vi "Get Addresses.vi"() -> (2 "Addresses":string[](array[string]), 3 "IP Addresses":T1[](array[typedef]) {"MAC U64" format="%012x"; "Mask" format="%08x"; "Address" format="%08x"})   [LabVIEW 2021, in "Networking_CIF_U.lvlib"]
doc: "Get the IPV4 address and subnet mask, the MAC address, and the resource description for all adaptors on the system. \n\nThe address list is filtered to only include valid IPV4 addresses with a valid MAC address. \n\nThis uses standard Windows and Linux system calls and parses the response."
uses:
  Networking_CIF_U.lvlib
  Typedef/IPV4 Address.ctl
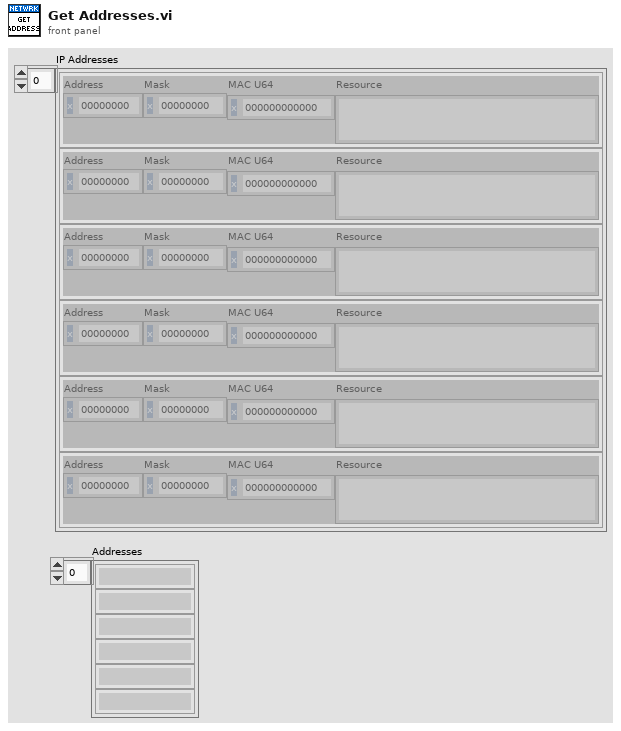
[diagram p1: front panel]
types:
  T1 = typedef "Networking_CIF_U.lvlib/IPV4 Address.ctl" = cluster{"Address":u32, "Mask":u32, "MAC U64":u64, "Resource":string}
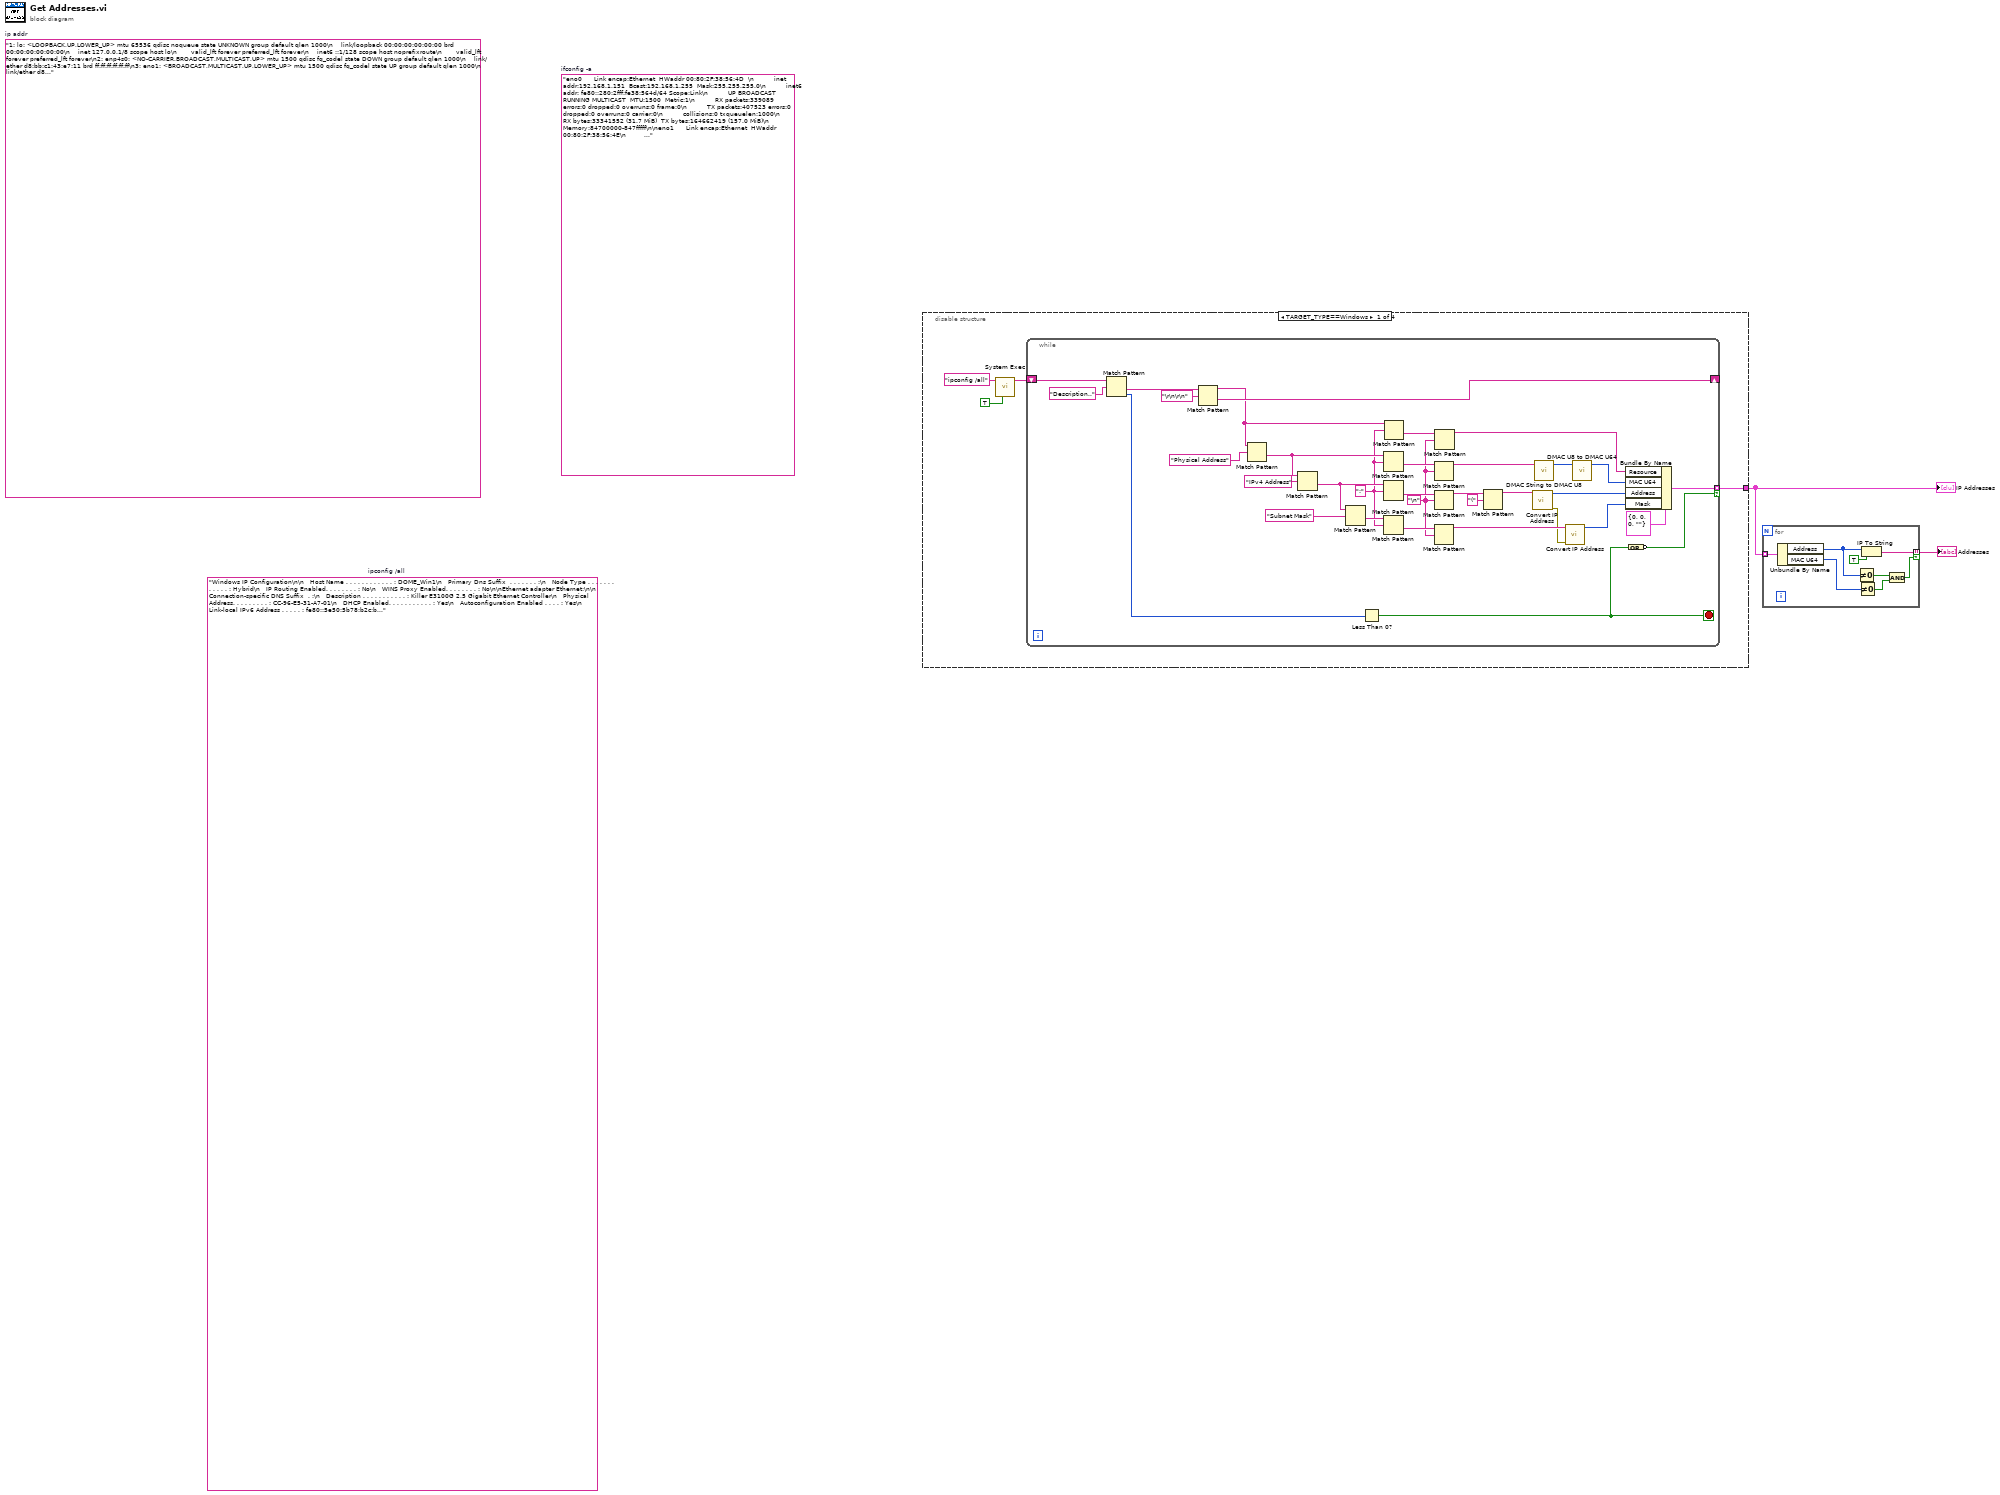
[diagram p0: block diagram]
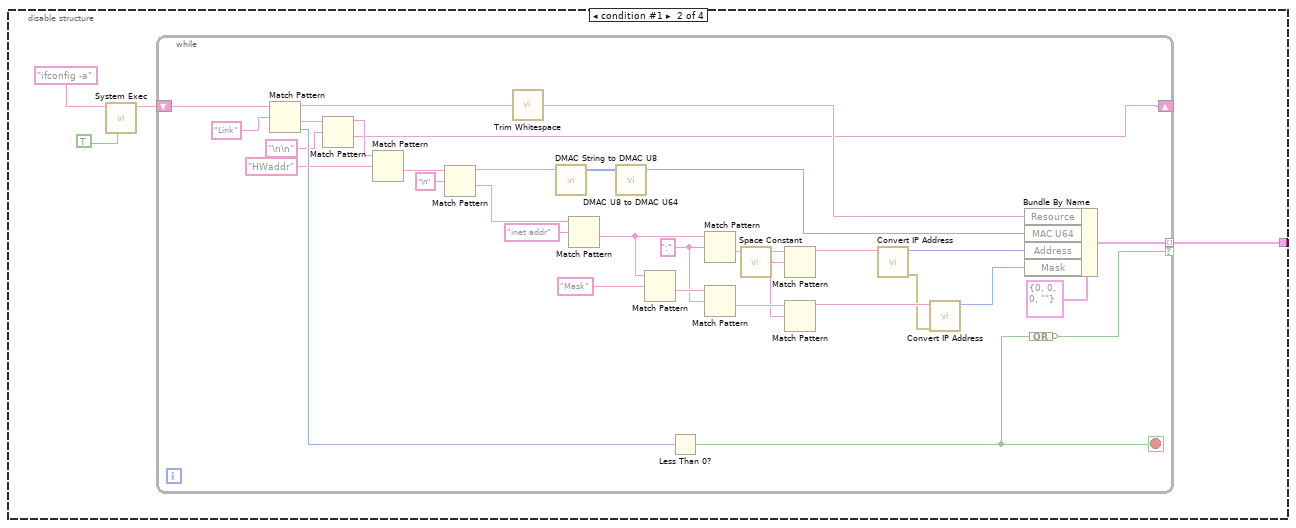
[diagram p2: hidden frame]
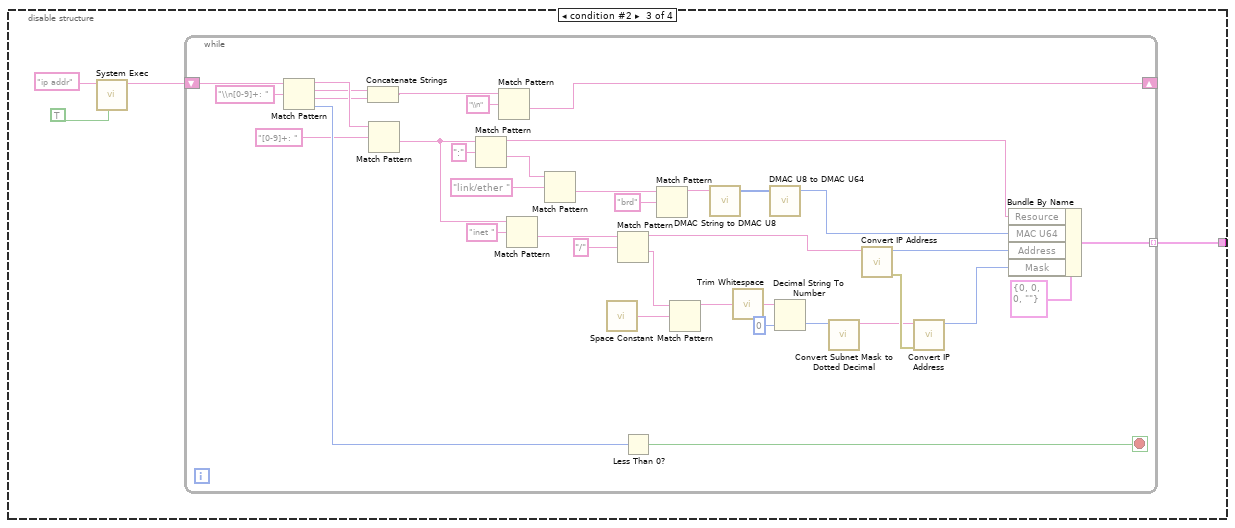
[diagram p3: hidden frame]
diagram:
  (unwired) "Windows IP Configuration\n\n   Host Name . . . . . . . . . . . . : DOME_Win1\n   Primary Dns Suffix  . . . . . . . :\n   Node Type . . . . . . . . . . . . : Hybrid\n   IP Routing Enabled. . . . . . . . : No\n   WINS Proxy Enabled. . . . . . . . : No\n\nEthernet adapter Ethernet:\n\n   Connection-specific DNS Suffix  . :\n   Description . . . . . . . . . . . : Killer E3100G 2.5 Gigabit Ethernet Controller\n   Physical Address. . . . . . . . . : CC-96-E5-31-A7-01\n   DHCP Enabled. . . . . . . . . . . : Yes\n   Autoconfiguration Enabled . . . . : Yes\n   Link-local IPv6 Address . . . . . : fe80::5e50:5b78:b2c:bb23%16(Preferred)\n   IPv4 Address. . . . . . . . . . . : 192.168.1.118(Preferred)\n   Subnet Mask . . . . . . . . . . . : 255.255.255.0\n   Lease Obtained. . . . . . . . . . : Monday, December 1, 2025 1:30:17 PM\n   Lease Expires . . . . . . . . . . : Sunday, January 10, 2162 1:38:58 AM\n   Default Gateway . . . . . . . . . : 192.168.1.1\n   DHCP Server . . . . . . . . . . . : 192.168.1.1\n   DHCPv6 IAID . . . . . . . . . . . : 114071269\n   DHCPv6 Client DUID. . . . . . . . : 00-01-00-01-2C-F9-5E-4C-CC-96-E5-31-A7-01\n   DNS Servers . . . . . . . . . . . : 208.67.222.123\n                                       208.67.220.123\n   NetBIOS over Tcpip. . . . . . . . : Enabled\n\nWireless LAN adapter Wi-Fi:\n\n   Media State . . . . . . . . . . . : Media disconnected\n   Connection-specific DNS Suffix  . :\n   Description . . . . . . . . . . . : Killer(R) Wi-Fi 6E AX1675i 160MHz Wireless Network Adapter (211NGW)\n   Physical Address. . . . . . . . . : 8C-17-59-A9-DC-15\n   DHCP Enabled. . . . . . . . . . . : Yes\n   Autoconfiguration Enabled . . . . : Yes\n\nWireless LAN adapter Local Area Connection* 1:\n\n   Media State . . . . . . . . . . . : Media disconnected\n   Connection-specific DNS Suffix  . :\n   Description . . . . . . . . . . . : Microsoft Wi-Fi Direct Virtual Adapter\n   Physical Address. . . . . . . . . : 8C-17-59-A9-DC-16\n   DHCP Enabled. . . . . . . . . . . : Yes\n   Autoconfiguration Enabled . . . . : Yes\n\nWireless LAN adapter Local Area Connection* 2:\n\n   Media State . . . . . . . . . . . : Media disconnected\n   Connection-specific DNS Suffix  . :\n   Description . . . . . . . . . . . : Microsoft Wi-Fi Direct Virtual Adapter #2\n   Physical Address. . . . . . . . . : 8E-17-59-A9-DC-15\n   DHCP Enabled. . . . . . . . . . . : Yes\n   Autoconfiguration Enabled . . . . : Yes\n\nEthernet adapter VMware Network Adapter VMnet1:\n\n   Connection-specific DNS Suffix  . :\n   Description . . . . . . . . . . . : VMware Virtual Ethernet Adapter for VMnet1\n   Physical Address. . . . . . . . . : 00-50-56-C0-00-01\n   DHCP Enabled. . . . . . . . . . . : Yes\n   Autoconfiguration Enabled . . . . : Yes\n   Link-local IPv6 Address . . . . . : fe80::dc23:c337:5224:768b%14(Preferred)\n   IPv4 Address. . . . . . . . . . . : 192.168.116.1(Preferred)\n   Subnet Mask . . . . . . . . . . . : 255.255.255.0\n   Lease Obtained. . . . . . . . . . : Monday, December 1, 2025 1:30:14 PM\n   Lease Expires . . . . . . . . . . : Wednesday, December 3, 2025 7:28:46 PM\n   Default Gateway . . . . . . . . . :\n   DHCP Server . . . . . . . . . . . : 192.168.116.254\n   DHCPv6 IAID . . . . . . . . . . . : 822104150\n   DHCPv6 Client DUID. . . . . . . . : 00-01-00-01-2C-F9-5E-4C-CC-96-E5-31-A7-01\n   NetBIOS over Tcpip. . . . . . . . : Enabled\n\nEthernet adapter VMware Network Adapter VMnet8:\n\n   Connection-specific DNS Suffix  . :\n   Description . . . . . . . . . . . : VMware Virtual Ethernet Adapter for VMnet8\n   Physical Address. . . . . . . . . : 00-50-56-C0-00-08\n   DHCP Enabled. . . . . . . . . . . : Yes\n   Autoconfiguration Enabled . . . . : Yes\n   Link-local IPv6 Address . . . . . : fe80::ac10:2aab:234a:a114%4(Preferred)\n   IPv4 Address. . . . . . . . . . . : 192.168.153.1(Preferred)\n   Subnet Mask . . . . . . . . . . . : 255.255.255.0\n   Lease Obtained. . . . . . . . . . : Monday, December 1, 2025 1:30:17 PM\n   Lease Expires . . . . . . . . . . : Wednesday, December 3, 2025 7:28:46 PM\n   Default Gateway . . . . . . . . . :\n   DHCP Server . . . . . . . . . . . : 192.168.153.254\n   DHCPv6 IAID . . . . . . . . . . . : 855658582\n   DHCPv6 Client DUID. . . . . . . . : 00-01-00-01-2C-F9-5E-4C-CC-96-E5-31-A7-01\n   Primary WINS Server . . . . . . . : 192.168.153.2\n   NetBIOS over Tcpip. . . . . . . . : Enabled\n\nEthernet adapter Bluetooth Network Connection:\n\n   Media State . . . . . . . . . . . : Media disconnected\n   Connection-specific DNS Suffix  . :\n   Description . . . . . . . . . . . : Bluetooth Device (Personal Area Network)\n   Physical Address. . . . . . . . . : 8C-17-59-A9-DC-19\n   DHCP Enabled. . . . . . . . . . . : Yes\n   Autoconfiguration Enabled . . . . : Yes"  # ipconfig /all
  (unwired) "eno0      Link encap:Ethernet  HWaddr 00:80:2F:38:56:4D  \n          inet addr:192.168.1.151  Bcast:192.168.1.255  Mask:255.255.255.0\n          inet6 addr: fe80::280:2fff:fe38:564d/64 Scope:Link\n          UP BROADCAST RUNNING MULTICAST  MTU:1500  Metric:1\n          RX packets:339089 errors:0 dropped:0 overruns:0 frame:0\n          TX packets:407523 errors:0 dropped:0 overruns:0 carrier:0\n          collisions:0 txqueuelen:1000\n          RX bytes:33341552 (31.7 MiB)  TX bytes:164662419 (157.0 MiB)\n          Memory:84700000-847fffff\n\neno1      Link encap:Ethernet  HWaddr 00:80:2F:38:56:4E\n          UP BROADCAST MULTICAST  MTU:1500  Metric:1\n          RX packets:0 errors:0 dropped:0 overruns:0 frame:0\n          TX packets:0 errors:0 dropped:0 overruns:0 carrier:0\n          collisions:0 txqueuelen:1000\n          RX bytes:0 (0.0 B)  TX bytes:0 (0.0 B)\n          Memory:84a00000-84afffff\n\nenp19s0f0 Link encap:Ethernet  HWaddr 08:C0:EB:46:0E:84\n          UP BROADCAST MULTICAST  MTU:1500  Metric:1\n          RX packets:0 errors:0 dropped:0 overruns:0 frame:0\n          TX packets:0 errors:0 dropped:0 overruns:0 carrier:0\n          collisions:0 txqueuelen:1000\n          RX bytes:0 (0.0 B)  TX bytes:0 (0.0 B)\n\nenp19s0f1 Link encap:Ethernet  HWaddr 08:C0:EB:46:0E:85\n          inet addr:192.168.12.2  Bcast:192.168.12.255  Mask:255.255.255.0\n          inet6 addr: fe80::ac0:ebff:fe46:e85/64 Scope:Link\n          UP BROADCAST RUNNING MULTICAST  MTU:1500  Metric:1\n          RX packets:283252 errors:0 dropped:0 overruns:0 frame:0\n          TX packets:61426 errors:0 dropped:0 overruns:0 carrier:0\n          collisions:0 txqueuelen:1000\n          RX bytes:355620193 (339.1 MiB)  TX bytes:16833550 (16.0 MiB)\n\nlo        Link encap:Local Loopback\n          inet addr:127.0.0.1  Mask:255.0.0.0\n          inet6 addr: ::1/128 Scope:Host\n          UP LOOPBACK RUNNING  MTU:65536  Metric:1\n          RX packets:134558 errors:0 dropped:0 overruns:0 frame:0\n          TX packets:134558 errors:0 dropped:0 overruns:0 carrier:0\n          collisions:0 txqueuelen:1000\n          RX bytes:11949346 (11.3 MiB)  TX bytes:11949346 (11.3 MiB)"  # ifconfig -a
  (unwired) "1: lo: <LOOPBACK,UP,LOWER_UP> mtu 65536 qdisc noqueue state UNKNOWN group default qlen 1000\n    link/loopback 00:00:00:00:00:00 brd 00:00:00:00:00:00\n    inet 127.0.0.1/8 scope host lo\n       valid_lft forever preferred_lft forever\n    inet6 ::1/128 scope host noprefixroute\n       valid_lft forever preferred_lft forever\n2: enp4s0: <NO-CARRIER,BROADCAST,MULTICAST,UP> mtu 1500 qdisc fq_codel state DOWN group default qlen 1000\n    link/ether d8:bb:c1:43:e7:11 brd ff:ff:ff:ff:ff:ff\n3: eno1: <BROADCAST,MULTICAST,UP,LOWER_UP> mtu 1500 qdisc fq_codel state UP group default qlen 1000\n    link/ether d8:bb:c1:43:e7:10 brd ff:ff:ff:ff:ff:ff\n    altname enp0s31f6\n    inet 192.168.1.242/24 brd 192.168.1.255 scope global noprefixroute eno1\n       valid_lft forever preferred_lft forever\n    inet6 fe80::dabb:c1ff:fe43:e710/64 scope link\n       valid_lft forever preferred_lft forever\n4: enp23s0f0np0: <NO-CARRIER,BROADCAST,MULTICAST,UP> mtu 1500 qdisc mq state DOWN group default qlen 1000\n    link/ether 04:3f:72:bd:14:a2 brd ff:ff:ff:ff:ff:ff\n5: enp23s0f1np1: <NO-CARRIER,BROADCAST,MULTICAST,UP> mtu 1500 qdisc mq state DOWN group default qlen 1000\n    link/ether 04:3f:72:bd:14:a3 brd ff:ff:ff:ff:ff:ff\n7: docker0: <NO-CARRIER,BROADCAST,MULTICAST,UP> mtu 1500 qdisc noqueue state DOWN group default\n    link/ether 8a:5f:4f:9d:9b:22 brd ff:ff:ff:ff:ff:ff\n    inet 172.17.0.1/16 brd 172.17.255.255 scope global docker0\n       valid_lft forever preferred_lft forever\n    inet6 fe80::885f:4fff:fe9d:9b22/64 scope link\n       valid_lft forever preferred_lft forever\n2022: br-b6147a662842: <BROADCAST,MULTICAST,UP,LOWER_UP> mtu 1500 qdisc noqueue state UP group default\n    link/ether e6:81:36:eb:4b:75 brd ff:ff:ff:ff:ff:ff\n    inet 172.18.0.1/16 brd 172.18.255.255 scope global br-b6147a662842\n       valid_lft forever preferred_lft forever\n    inet6 fe80::e481:36ff:feeb:4b75/64 scope link\n       valid_lft forever preferred_lft forever\n2025: veth8e9c1bb@if2: <BROADCAST,MULTICAST,UP,LOWER_UP> mtu 1500 qdisc noqueue master br-b6147a662842 state UP group default\n    link/ether 66:7b:84:4d:96:ba brd ff:ff:ff:ff:ff:ff link-netnsid 0\n    inet6 fe80::647b:84ff:fe4d:96ba/64 scope link\n       valid_lft forever preferred_lft forever\n2026: veth719d540@if2: <BROADCAST,MULTICAST,UP,LOWER_UP> mtu 1500 qdisc noqueue master br-b6147a662842 state UP group default\n    link/ether 4e:3e:af:11:6f:2c brd ff:ff:ff:ff:ff:ff link-netnsid 1\n    inet6 fe80::4c3e:afff:fe11:6f2c/64 scope link\n       valid_lft forever preferred_lft forever\n2034: br-e29f2d474aae: <NO-CARRIER,BROADCAST,MULTICAST,UP> mtu 1500 qdisc noqueue state DOWN group default\n    link/ether 76:6d:e5:b8:89:b4 brd ff:ff:ff:ff:ff:ff\n    inet 172.19.0.1/16 brd 172.19.255.255 scope global br-e29f2d474aae\n       valid_lft forever preferred_lft forever\n    inet6 fe80::746d:e5ff:feb8:89b4/64 scope link\n       valid_lft forever preferred_lft forever"  # ip addr
  n1 = disable-structure shown="TARGET_TYPE==Windows" {
    disable-tunnel: [w3 w41 w79 _] -> w2
    frame condition #0 (active) {
      n2 = call <vilib>:"System Exec.vi"("run minimized? (F)"=TRUE, "command line"="ipconfig /all") -> ("standard output"=w4:string)  [unwired: 6 in, 3 out]
      n3 = while {
        shift-right: [w12] -> _
        shift-left: w4 -> [w17]
        tunnel: [w28] -> w3 mode=indexing if=w27
        stop <- w29 stop-if-true
        w9 = "\n"
        w10 = ":" ("regular expression")
        n4 = Match Pattern(string=w17, regular expression="Description..") -> (after substring=w14:string, offset past match=w15:i32)  [unwired: 1 in, 2 out]
        n5 = Match Pattern(string=w14, regular expression="\r\n\r\n") -> (before substring=w8:string, after substring=w12:string)  [unwired: 1 in, 2 out]
        n6 = Match Pattern(string=w8, regular expression="Physical Address") -> (after substring=w24:string)  [unwired: 1 in, 3 out]
        n7 = Match Pattern(string=w24, regular expression="IPv4 Address") -> (after substring=w38:string)  [unwired: 1 in, 3 out]
        n8 = Match Pattern(string=w38, regular expression="Subnet Mask") -> (after substring=w37:string)  [unwired: 1 in, 3 out]
        n9 = Less Than 0?(x=w15) -> (x < 0?=w29:bool)
        n10 = Match Pattern(string=w24, regular expression=w10) -> (after substring=w25:string)  [unwired: 1 in, 3 out]
        n11 = Match Pattern(string=w38, regular expression=w10) -> (after substring=w36:string)  [unwired: 1 in, 3 out]
        n12 = Match Pattern(string=w37, regular expression=w10) -> (after substring=w35:string)  [unwired: 1 in, 3 out]
        n13 = Match Pattern(string=w8, regular expression=w10) -> (after substring=w11:string)  [unwired: 1 in, 3 out]
        n14 = Match Pattern(string=w25, regular expression=w9) -> (before substring=w23:string)  [unwired: 1 in, 3 out]
        n15 = Match Pattern(string=w36, regular expression=w9) -> (before substring=w20:string)  [unwired: 1 in, 3 out]
        n16 = Match Pattern(string=w35, regular expression=w9) -> (before substring=w34:string)  [unwired: 1 in, 3 out]
        n17 = Match Pattern(string=w11, regular expression=w9) -> (before substring=w7:string)  [unwired: 1 in, 3 out]
        n18 = Match Pattern(string=w20, regular expression="(") -> (before substring=w19:string)  [unwired: 1 in, 3 out]
        n19 = call "Convert IP Address.vi"("IP"=w19) -> ("error out"=w33:errorcluster, "net address"=w31:u32)  [unwired: 9 in]
        n20 = call "DMAC String to DMAC U8.vi"("DMAC String"=w23) -> ("DestinationMACAddress"=w22:u8[])  [unwired: 4 in]
        n21 = call "Convert IP Address.vi"("error in (no error)"=w33, "IP"=w34) -> ("net address"=w30:u32)  [unwired: 8 in, 1 out]
        n22 = call "DMAC U8 to DMAC U64.vi"("DestinationMACAddress"=w22) -> ("DMAC U64"=w21:u64)  [unwired: 4 in]
        n23 = Bundle By Name(cluster=T1 {"Address"=0, "Mask"=0, "MAC U64"=0, "Resource"=""} ("IPV4 Address"), "Resource"=w7, "MAC U64"=w21, "Address"=w31, "Mask"=w30) -> (w28:T1)
        n24 = Compound Arithmetic op=OR(w29) -> (invert w27:bool)
      }
    }
    frame condition #1 {
      n25 = call <vilib>:"System Exec.vi"("run minimized? (F)"=TRUE, "command line"="ifconfig -a") -> ("standard output"=w42:string)  [unwired: 6 in, 3 out]
      n26 = while {
        shift-right: [w47] -> _
        shift-left: w42 -> [w45]
        tunnel: [w62] -> w41 mode=indexing if=w61
        stop <- w63 stop-if-true
        w73 = ":" ("regular expression")
        n27 = Match Pattern(string=w45, regular expression="Link") -> (before substring=w50:string, after substring=w49:string, offset past match=w60:i32)  [unwired: 1 in, 1 out]
        n28 = Match Pattern(string=w49, regular expression="\n\n") -> (before substring=w48:string, after substring=w47:string)  [unwired: 1 in, 2 out]
        n29 = Match Pattern(string=w48, regular expression="HWaddr") -> (after substring=w56:string)  [unwired: 1 in, 3 out]
        n30 = Match Pattern(string=w56, regular expression="\n") -> (before substring=w52:string, after substring=w55:string)  [unwired: 1 in, 2 out]
        n31 = call <vilib>:"Trim Whitespace.vi"("string"=w50) -> ("trimmed string"=w58:string)  [unwired: 1 in]
        n32 = call "DMAC String to DMAC U8.vi"("DMAC String"=w52) -> ("DestinationMACAddress"=w53:u8[])  [unwired: 4 in]
        n33 = Match Pattern(string=w55, regular expression="inet addr") -> (after substring=w75:string)  [unwired: 1 in, 3 out]
        n34 = call "DMAC U8 to DMAC U64.vi"("DestinationMACAddress"=w53) -> ("DMAC U64"=w51:u64)  [unwired: 4 in]
        n35 = Match Pattern(string=w75, regular expression="Mask") -> (after substring=w74:string)  [unwired: 1 in, 3 out]
        n36 = Less Than 0?(x=w60) -> (x < 0?=w63:bool)
        n37 = Match Pattern(string=w75, regular expression=w73) -> (after substring=w72:string)  [unwired: 1 in, 3 out]
        n38 = Match Pattern(string=w74, regular expression=w73) -> (after substring=w71:string)  [unwired: 1 in, 3 out]
        n39 = call <vilib>:"Space Constant.vi"() -> ("String"=w70:string)
        n40 = Match Pattern(string=w72, regular expression=w70) -> (before substring=w69:string)  [unwired: 1 in, 3 out]
        n41 = Match Pattern(string=w71, regular expression=w70) -> (before substring=w68:string)  [unwired: 1 in, 3 out]
        n42 = call "Convert IP Address.vi"("IP"=w69) -> ("error out"=w67:errorcluster, "net address"=w65:u32)  [unwired: 9 in]
        n43 = call "Convert IP Address.vi"("error in (no error)"=w67, "IP"=w68) -> ("net address"=w64:u32)  [unwired: 8 in, 1 out]
        n44 = Bundle By Name(cluster=T1 {"Address"=0, "Mask"=0, "MAC U64"=0, "Resource"=""} ("IPV4 Address"), "Resource"=w58, "MAC U64"=w51, "Address"=w65, "Mask"=w64) -> (w62:T1)
        n45 = Compound Arithmetic op=OR(w63) -> (invert w61:bool)
      }
    }
    frame condition #2 {
      n46 = call <vilib>:"System Exec.vi"("run minimized? (F)"=TRUE, "command line"="ip addr") -> ("standard output"=w78:string)  [unwired: 6 in, 3 out]
      n47 = while {
        shift-right: [w93] -> _
        shift-left: w78 -> [w100]
        tunnel: [w109] -> w79 mode=indexing
        stop <- w110 stop-if-true
        n48 = Match Pattern(string=w100, regular expression="\\n[0-9]+: ") -> (before substring=w98:string, match substring=w97:string, after substring=w96:string, offset past match=w99:i32)  [unwired: 1 in]
        n49 = Concatenate Strings(w97, w96) -> (w95:string)
        n50 = Match Pattern(string=w98, regular expression="[0-9]+: ") -> (after substring=w91:string)  [unwired: 1 in, 3 out]
        n51 = Match Pattern(string=w91, regular expression=":") -> (before substring=w89:string, after substring=w88:string)  [unwired: 1 in, 2 out]
        n52 = Match Pattern(string=w95, regular expression="\\n") -> (after substring=w93:string)  [unwired: 1 in, 3 out]
        n53 = Match Pattern(string=w91, regular expression="inet ") -> (after substring=w117:string)  [unwired: 1 in, 3 out]
        n54 = Match Pattern(string=w88, regular expression="link/ether ") -> (after substring=w84:string)  [unwired: 1 in, 3 out]
        n55 = call <vilib>:"Space Constant.vi"() -> ("String"=w115:string)
        n56 = Match Pattern(string=w117, regular expression="/") -> (before substring=w103:string, after substring=w108:string)  [unwired: 1 in, 2 out]
        n57 = Less Than 0?(x=w99) -> (x < 0?=w110:bool)
        n58 = Match Pattern(string=w84, regular expression="brd") -> (before substring=w83:string)  [unwired: 1 in, 3 out]
        n59 = Match Pattern(string=w108, regular expression=w115) -> (before substring=w107:string)  [unwired: 1 in, 3 out]
        n60 = call "DMAC String to DMAC U8.vi"("DMAC String"=w83) -> ("DestinationMACAddress"=w82:u8[])  [unwired: 4 in]
        n61 = call <vilib>:"Trim Whitespace.vi"("string"=w107) -> ("trimmed string"=w106:string)  [unwired: 1 in]
        n62 = call "DMAC U8 to DMAC U64.vi"("DestinationMACAddress"=w82) -> ("DMAC U64"=w85:u64)  [unwired: 4 in]
        n63 = Decimal String To Number(string=w106, default (0L)=u8 0 ("default (0 I32)")) -> (number=w105:u8)  [unwired: 1 in, 1 out]
        n64 = call "Convert Subnet Mask to Dotted Decimal.vi"("Mask CIDR"=w105) -> ("Mask"=w102:string)  [unwired: 9 in, 1 out]
        n65 = call "Convert IP Address.vi"("IP"=w103) -> ("error out"=w114:errorcluster, "net address"=w112:u32)  [unwired: 9 in]
        n66 = call "Convert IP Address.vi"("error in (no error)"=w114, "IP"=w102) -> ("net address"=w111:u32)  [unwired: 8 in, 1 out]
        n67 = Bundle By Name(cluster=T1 {"Address"=0, "Mask"=0, "MAC U64"=0, "Resource"=""} ("IPV4 Address"), "Resource"=w89, "MAC U64"=w85, "Address"=w112, "Mask"=w111) -> (w109:T1)
      }
    }
    frame condition #3 {
    }
  }
  "IP Addresses" <- w2
  n68 = for {
    tunnel: w2 -> [w126] mode=indexing
    tunnel: [w124] -> w1 mode=indexing if=w119
    n69 = Unbundle By Name(w126) -> ("Address"=w123:u32, "MAC U64"=w122:u64)
    n70 = Not Equal To 0?(x=w123) -> (x != 0?=w121:bool)
    n71 = Not Equal To 0?(x=w122) -> (x != 0?=w120:bool)
    n72 = IP To String(1:TRUE ("dot notation? (F)"), 2:w123) -> (0:w124:string)
    n73 = Compound Arithmetic op=AND(w121, w120) -> (w119:bool)
  }
  "Addresses" <- w1
